vi "Fetch (Waveform).vi"(8 "error in (no error)":errorcluster, 9 "Maximum Time (10000ms)":u32=10000, 10 "Channel (0:Channel1)":u16(ring) items=["Channel1", "Channel2", "Channel3", "Channel4", "Math1", "Math2", "Math3", "Math3", "Reference1", "Reference2", "Reference3", "Reference4"], 11 "VISA resource name":refnum<visa-resource-name>) -> (0 "error out":errorcluster, 2 "Waveform Data":waveform(dbl)(graph)={"t0"=timestamp(3.694502999999883e-07 s since 1904-01-01), "dt"=5e-07, "Y"=array[10000 elements]}, 3 "VISA resource name out":refnum<visa-resource-name>)   [LabVIEW 2011, in "Tektronix 7000 Series.lvlib"]
doc: "Returns the waveform that an oscilloscope acquires for a channel you specify. An acquisition that you initiate before calling this VI generates the waveform.\n\nYou first enable channels with the Configure Channel VI. Then you use the Initiate VI to start an acquisition on the enabled channels. An oscilloscope concurrently acquires waveforms for these channels. You must call the Fetch Waveform VI separately to obtain waveforms for each enabled channel. However, you also can call the Read Waveform VI instead of using the above low-level VIs.\n\n<B>Note:</B> Use the Fetch Waveform VI only with other low-level VIs, such as the Initiate VI, the Abort VI, and the Fetch Waveform Measurement VI. High-level VIs such as the Read Waveform VI automatically incorporate the functions of the Initiate VI and the Fetch Waveform VI. The Fetch Waveform VI does not check the status of an instrument."
uses:
  Tektronix 7000 Series.lvlib
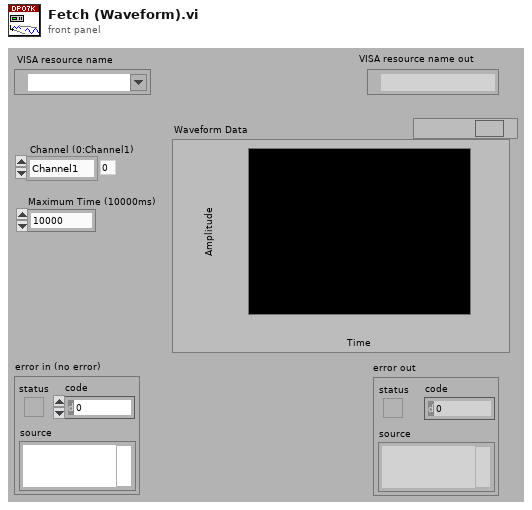
[diagram p1: front panel]
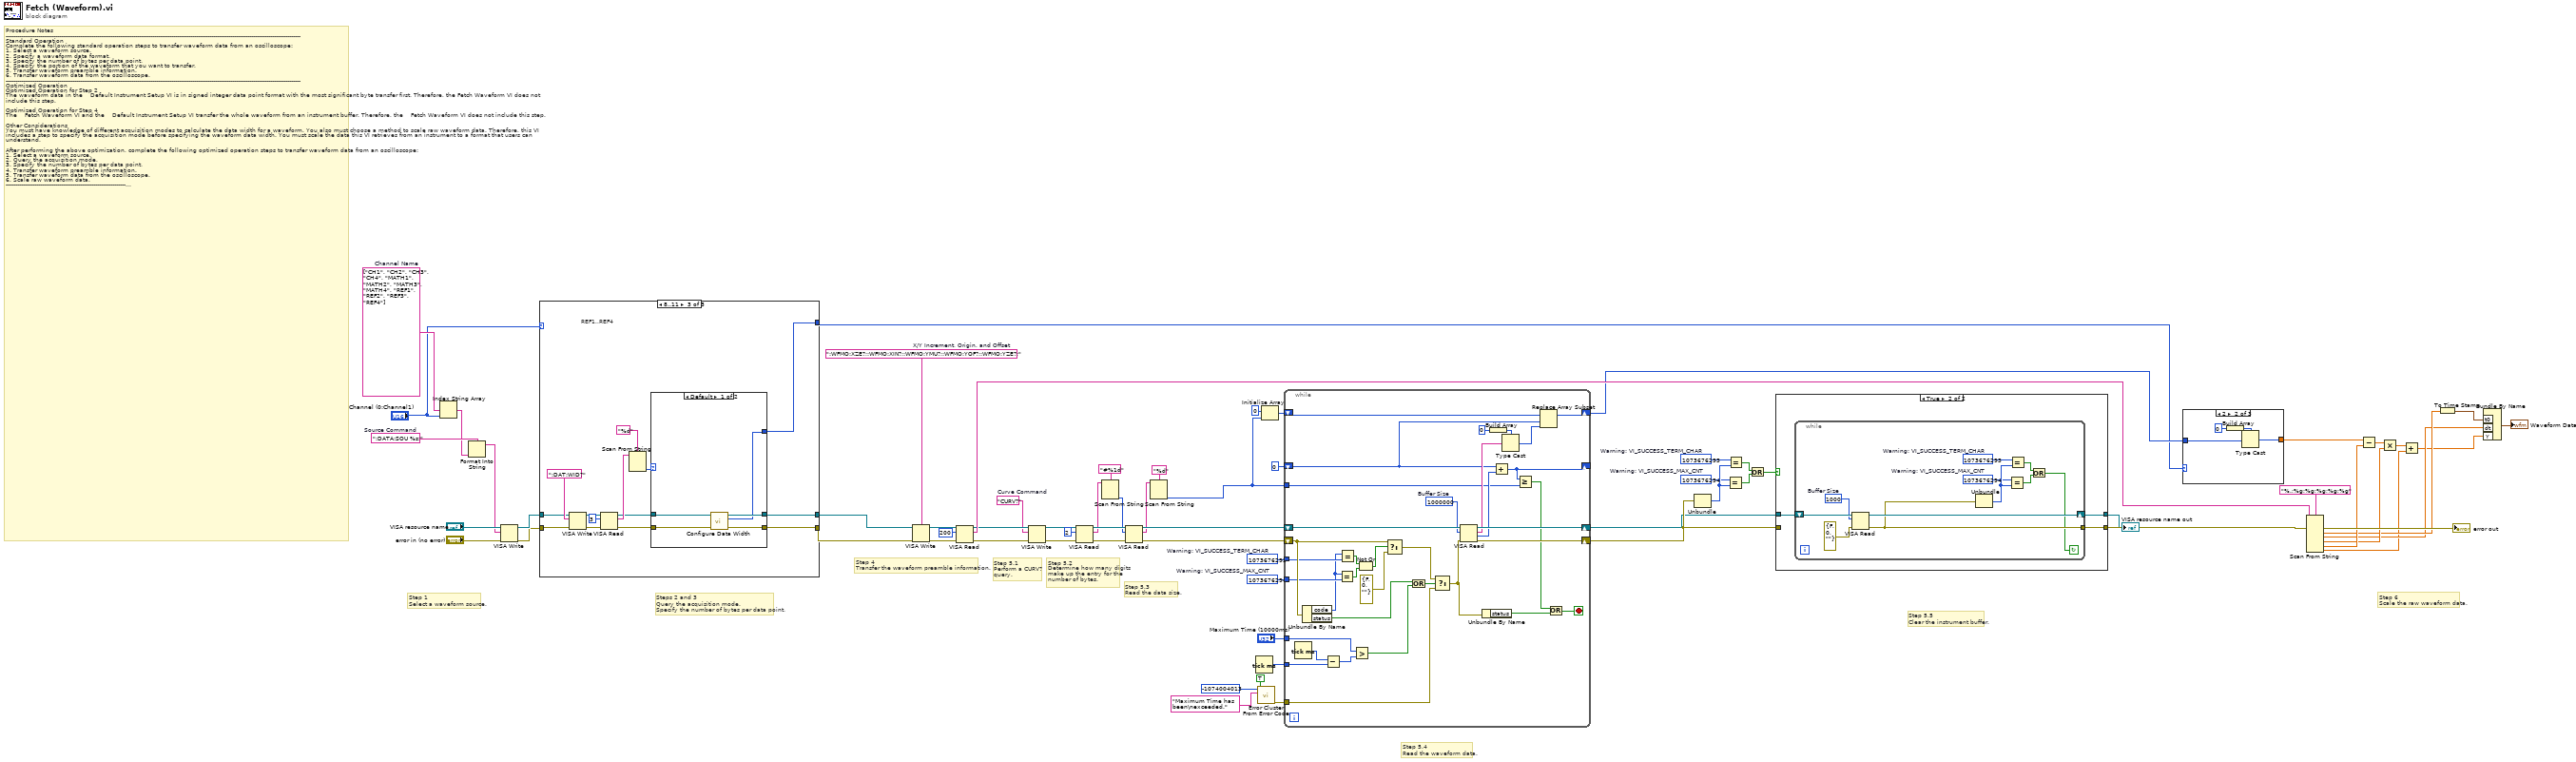
[diagram p0: block diagram]
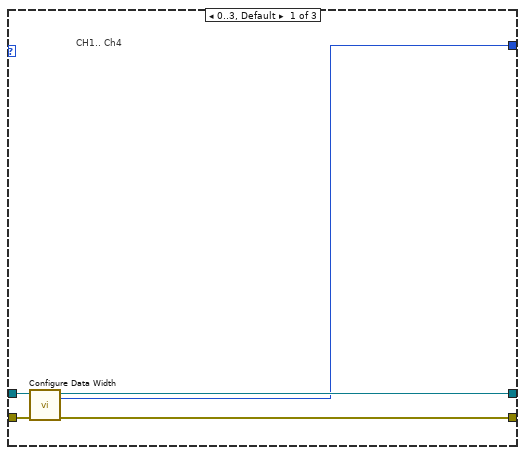
[diagram p2: hidden frame]
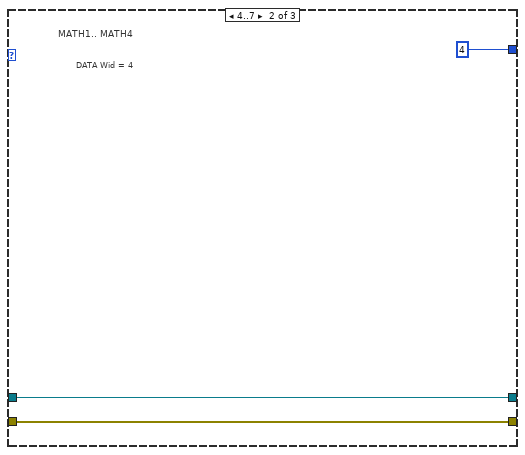
[diagram p3: hidden frame]
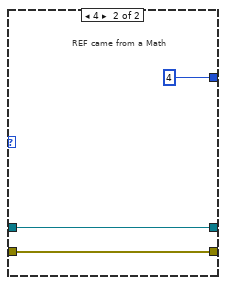
[diagram p4: hidden frame]
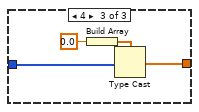
[diagram p6: hidden frame]
diagram:
  w11 = "CURV?"  # Curve Command
  w42 = string[] ["CH1", "CH2", "CH3", "CH4", "MATH1", "MATH2", "MATH3", "MATH4", "REF1", "REF2", "REF3", "REF4"]  # Channel Name
  w48 = 1073676294  # Warning: VI_SUCCESS_MAX_CNT
  w49 = 1073676293  # Warning: VI_SUCCESS_TERM_CHAR
  w52 = 1073676294  # Warning: VI_SUCCESS_MAX_CNT
  w51 = 1073676293  # Warning: VI_SUCCESS_TERM_CHAR
  w68 = ":DATA:SOU %s;"  # Source Command
  w37 = ":WFMO:XZE?;:WFMO:XIN?;:WFMO:YMU?;:WFMO:YOF?;:WFMO:YZE?;"  # X/Y Increment, Origin, and Offset
  # "Step 1       \nSelect a waveform source."
  # "Steps 2 and 3\nQuery the acquisition mode. \nSpecify the number of bytes per data point."
  # "Step 6    \nScale the raw waveform data."
  # "Step 5.5    \nClear the instrument buffer."
  # "Step 5.4   \nRead the waveform data."
  # "Step 5.3      \nRead the data size."
  # "Step 5.2      \nDetermine how many digits\nmake up the entry for the \nnumber of bytes."
  # "Step 5.1      \nPerform a CURV?\nquery."
  # "Step 4\nTransfer the waveform preamble information."
  # "Procedure Notes\n-----------------------------------------------------------------------------------------------------------------------------------------------------------\nStandard Operation\nComplete the following standard operation steps to transfer waveform data from an oscilloscope:\n1. Select a waveform source.\n2. Specify a waveform data format.\n3. Specify the number of bytes per data point.\n4. Specify the portion of the waveform that you want to transfer.\n5. Transfer waveform preamble information.\n6. Transfer waveform data from the oscilloscope.\n-----------------------------------------------------------------------------------------------------------------------------------------------------------\nOptimized Operation\nOptimized Operation for Step 2\nThe waveform data in the    Default Instrument Setup VI is in signed integer data point format with the most significant byte transfer first. Therefore, the Fetch Waveform VI does not include this step.\n\nOptimized Operation for Step 4 \nThe    Fetch Waveform VI and the    Default Instrument Setup VI transfer the whole waveform from an instrument buffer. Therefore, the    Fetch Waveform VI does not include this step.\n\nOther Considerations\nYou must have knowledge of different acquisition modes to calculate the data width for a waveform. You also must choose a method to scale raw waveform data. Therefore, this VI includes a step to specify the acquisition mode before specifying the waveform data width. You must scale the data this VI retrieves from an instrument to a format that users can understand.\n\nAfter performing the above optimization, complete the following optimized operation steps to transfer waveform data from an oscilloscope:\n1. Select a waveform source.\n2. Query the acquisition mode.\n3. Specify the number of bytes per data point.\n4. Transfer waveform preamble information.\n5. Transfer waveform data from the oscilloscope.\n6. Scale raw waveform data.\n-----------------------------------------------------------------------------------------------------------------------------------------------------------\nDetailed Steps\nThe following steps detail the behavior of this VI:\n1. Select a waveform source. \n2. Query and determine the acquisition mode. A correct determination is critical to steps 3 and 6.\n    -----------------------------------------------\n    Acquisition Mode |  Data Width   \n    -----------------------------------------------\n    Normal                       |   1                      \n    -----------------------------------------------\n    Peak Detect               |   1                      \n    -----------------------------------------------\n    Hi Res                        |   2                      \n    -----------------------------------------------\n    Envelope                   |   1                      \n    ----------------------------------------------- \n    Average                    |   2                      \n    -----------------------------------------------\n3. Specify the number of bytes per data point. For the Hi Res or Average acquisition modes, set the data width to 2. For all other acquisition modes, set the data width to 1.\n4. Transfer the waveform preamble information. Necessary preamble information includes XZero, XIncrement, YMultiplier, YOffset, and YZero. This VI uses XZero and XIncrement to configure the x-axis of output waveforms and uses YMultiplier, YOffset, and YZero to scale data values. This VI then parses the return string of the preamble query in step 6.\n5. Transfer waveform data from the oscilloscope.\n    5.1 Perform a CURV? query.\n    5.2 Determine how many digits make up the entry for the number of bytes.\n    5.3 Read the data size.\n    5.4 Call the VISA Read VI repeatedly with a buffer size of 10000 until you obtain as much data as the data size specifies. Use      an 8-bit array to store the raw waveform data you obtain. \n    5.5 Continue reading the data remaining in the instrument buffer until the buffer is empty.\n6. Scale the raw waveform data.\n    6.1 Cast the waveform data to a 16-bit array if the data width is 2. Split the waveform data into a minimum and a maximum data array if the acquisition mode is Peak Detect or Envelope. This VI skips this step if the data width is 1.\n    6.2 Parse the preamble information.\n    6.3 Scale the waveform data according to the following formula:\n          Data_Value_in_units = (Raw_Data_Value - YOffset) * YMultiplier + YZero\n          The resulting waveform data has a unit of volts.\n    6.4 Build a waveform graph."
  n1 = Index String Array(1:"Channel (0:Channel1)", 2:w42) -> (0:w67:string)  [unwired: 1 in]
  n2 = Format Into String(format string=w68, w67) -> (resulting string=w39:string)  [unwired: 2 in, 1 out]
  n3 = VISA Write(VISA resource name="VISA resource name", write buffer=w39, error in (no error)="error in (no error)") -> (VISA resource name out=w31:refnum<visa-resource-name>, error out=w30:errorcluster)  [unwired: 1 out]
  n4 = case shown="8..11" "Channel (0:Channel1)" {
    tunnel: w31 -> [w73 w76 w85]
    tunnel: w30 -> [w72 w75 w86]
    tunnel: [w71 w76 w79] -> w13
    tunnel: [w70 w75 w78] -> w12
    tunnel: [w69 u32 4 ("byte count") w77] -> w16
    frame 0..3, Default {
      # "CH1.. Ch4"
      n5 = call "Configure Data Width.vi"("error in (no error)"=w72, "VISA resource name"=w73) -> ("error out"=w70:errorcluster, "Width"=w69:i32, "VISA resource name out"=w71:refnum<visa-resource-name>)  [unwired: 7 in]
    }
    frame 4..7 {
      # "DATA Wid = 4"
      # "MATH1.. MATH4"
    }
    frame 8..11 {
      # "REF1..REF4"
      n6 = VISA Write(VISA resource name=w85, write buffer=":DAT:WID?", error in (no error)=w86) -> (VISA resource name out=w90:refnum<visa-resource-name>, error out=w89:errorcluster)  [unwired: 1 out]
      n7 = VISA Read(VISA resource name=w90, byte count=u32 3, error in (no error)=w89) -> (VISA resource name out=w81:refnum<visa-resource-name>, read buffer=w84:string, error out=w80:errorcluster)  [unwired: 1 out]
      n8 = Scan From String(format string="%d", input string=w84) -> (output 1=w82:i32)  [unwired: 3 in, 3 out]
      n9 = case shown="Default" w82 {
        tunnel: w81 -> [w95 w98]
        tunnel: w80 -> [w94 w97]
        tunnel: [w93 w98] -> w79
        tunnel: [w92 w97] -> w78
        tunnel: [w91 u32 4 ("byte count")] -> w77
        frame Default {
          n10 = call "Configure Data Width.vi"("error in (no error)"=w94, "VISA resource name"=w95) -> ("error out"=w92:errorcluster, "Width"=w91:i32, "VISA resource name out"=w93:refnum<visa-resource-name>)  [unwired: 7 in]
        }
        frame 4 {
          # "REF came from a Math"
        }
      }
    }
  }
  n11 = VISA Write(VISA resource name=w13, write buffer=w37, error in (no error)=w12) -> (VISA resource name out=w65:refnum<visa-resource-name>, error out=w64:errorcluster)  [unwired: 1 out]
  n12 = VISA Read(VISA resource name=w65, byte count=u32 200, error in (no error)=w64) -> (VISA resource name out=w29:refnum<visa-resource-name>, read buffer=w63:string, error out=w28:errorcluster)  [unwired: 1 out]
  n13 = VISA Write(VISA resource name=w29, write buffer=w11, error in (no error)=w28) -> (VISA resource name out=w1:refnum<visa-resource-name>, error out=w10:errorcluster)  [unwired: 1 out]
  n14 = VISA Read(VISA resource name=w1, byte count=u32 2, error in (no error)=w10) -> (VISA resource name out=w7:refnum<visa-resource-name>, read buffer=w5:string, error out=w6:errorcluster)  [unwired: 1 out]
  n15 = Scan From String(format string="#%1d", input string=w5) -> (output 1=w4:i32)  [unwired: 3 in, 3 out]
  n16 = VISA Read(VISA resource name=w7, byte count=w4, error in (no error)=w6) -> (VISA resource name out=w27:refnum<visa-resource-name>, read buffer=w2:string, error out=w26:errorcluster)  [unwired: 1 out]
  n17 = Scan From String(format string="%d", input string=w2) -> (output 1=w59:i32)  [unwired: 3 in, 3 out]
  n18 = Tick Count (ms)() -> (millisecond timer value=w19:u32)
  n19 = call <vilib>:"Error Cluster From Error Code.vi"("show call chain? (False)"=TRUE, "error message (\"\")"="Maximum Time has been\nexceeded." ("error message (\"\")"), "error code (0)"=-1074004013) -> ("error out"=w17:errorcluster)  [unwired: 6 in]
  n20 = Initialize Array(i8 0 ("element"), w59) -> (w57:i8[])
  n21 = while {
    shift-right: [w131] -> w14
    shift-left: w27 -> [w133]
    shift-right: [w130] -> w15
    shift-left: w26 -> [w119]
    shift-right: [w126] -> w47
    shift-left: w57 -> [w127]
    tunnel: w59 -> [w123]
    shift-right: [w120] -> _
    shift-left: 0 -> [w121]
    tunnel: w49 -> [w118]
    tunnel: w48 -> [w117]
    tunnel: w19 -> [w111]
    tunnel: "Maximum Time (10000ms)" -> [w110]
    tunnel: w17 -> [w105]
    stop <- w101 stop-if-true
    w132 = 1000000  # Buffer Size
    n22 = Tick Count (ms)() -> (millisecond timer value=w112:u32)
    n23 = Unbundle By Name(w119) -> ("code"=w116:i32, "status"=w104:bool)
    n24 = Subtract(x=w112, y=w111) -> (x-y=w109:u32)
    n25 = Equal?(x=w116, y=w117) -> (x = y?=w114:bool)
    n26 = Equal?(x=w116, y=w118) -> (x = y?=w115:bool)
    n27 = Greater?(x=w110, y=w109) -> (0:w103:bool)
    n28 = Not Or(1:w114, 2:w115) -> (0:w113:bool)
    n29 = Select(t=w119, s=w113, f=errorcluster {"status"=FALSE, "code"=0, "source"=""} ("error in (no error)")) -> (s? t:f=w106:errorcluster)
    n30 = Or(x=w104, y=w103) -> (x .or. y?=w107:bool)
    n31 = Select(t=w106, s=w107, f=w105) -> (s? t:f=w100:errorcluster)
    n32 = VISA Read(VISA resource name=w133, byte count=w132, error in (no error)=w100) -> (VISA resource name out=w131:refnum<visa-resource-name>, read buffer=w125:string, return count=w124:u32, error out=w130:errorcluster)
    n33 = Unbundle By Name(w100) -> ("status"=w99:bool)
    n34 = Build Array(i8 0) -> (w129:i8[])
    n35 = Add(x=w121, y=w124) -> (x+y=w120:u32)
    n36 = Type Cast(type=w129, x=w125) -> (*(type *) &x=w122:i8[])
    n37 = Greater Or Equal?(x=w120, y=w123) -> (x >= y?=w102:bool)
    n38 = Replace Array Subset(array=w127, new element=w122, index=w121) -> (w126:i8[])
    n39 = Or(x=w102, y=w99) -> (x .or. y?=w101:bool)
  }
  n40 = Unbundle(w15) -> ("code"=w53:i32)  [unwired: 2 out]
  n41 = Equal?(x=w52, y=w53) -> (x = y?=w55:bool)
  n42 = Equal?(x=w51, y=w53) -> (x = y?=w56:bool)
  n43 = Or(x=w56, y=w55) -> (x .or. y?=w54:bool)
  n44 = case shown="True" w54 {
    tunnel: w14 -> [w135 w138]
    tunnel: w15 -> [w134 _]
    tunnel: [w135 w137] -> w60
    tunnel: [w134 w136] -> w62
    frame False {
    }
    frame True {
      n45 = while {
        shift-right: [w148] -> w137
        shift-left: w138 -> [w149]
        tunnel: [w141] -> w136
        stop <- w140 continue-if-true
        w143 = 1073676294  # Warning: VI_SUCCESS_MAX_CNT
        w142 = 1073676293  # Warning: VI_SUCCESS_TERM_CHAR
        w147 = u32 1000  # Buffer Size
        n46 = VISA Read(VISA resource name=w149, byte count=w147, error in (no error)=errorcluster {"status"=FALSE, "code"=0, "source"=""}) -> (VISA resource name out=w148:refnum<visa-resource-name>, error out=w141:errorcluster)  [unwired: 2 out]
        n47 = Unbundle(w141) -> ("code"=w144:i32)  [unwired: 2 out]
        n48 = Equal?(x=w143, y=w144) -> (x = y?=w145:bool)
        n49 = Equal?(x=w142, y=w144) -> (x = y?=w146:bool)
        n50 = Or(x=w146, y=w145) -> (x .or. y?=w140:bool)
      }
    }
  }
  "VISA resource name out" <- w60
  n51 = case shown="2" w16 {
    tunnel: w47 -> [w150 w152 w156]
    tunnel: [w150 w151 w155] -> w35
    frame 1, Default {
    }
    frame 2 {
      n52 = Build Array(i16 0 ("element")) -> (w153:i16[])
      n53 = Type Cast(type=w153, x=w152) -> (*(type *) &x=w151:i16[])
    }
    frame 4 {
      n54 = Build Array(sgl 0.0 ("element")) -> (w157:sgl[])
      n55 = Type Cast(type=w157, x=w156) -> (*(type *) &x=w155:sgl[])
    }
  }
  n56 = Scan From String(format string="%.;%g;%g;%g;%g;%g", input string=w63, error in=w62) -> (error out=→"error out":errorcluster, output 1=w34:dbl, output 2=w32:dbl, output 3=w43:dbl, output 4=w44:dbl, output 5=w24:dbl)  [unwired: 6 in, 2 out]
  n57 = Subtract(x=w35, y=w44) -> (x-y=w45:dbl[])
  n58 = Multiply(x=w45, y=w43) -> (x*y=w25:dbl[])
  n59 = Add(x=w25, y=w24) -> (x+y=w23:dbl[])
  n60 = To Time Stamp(1:w34) -> (0:w33:timestamp)
  n61 = Bundle By Name ("Build Waveform")("t0"=w33, "dt"=w32, "Y"=w23) -> (→"Waveform Data":waveform(dbl))  [unwired: 1 in]
